vi "XYStage.TestLauncher.vi"() -> ()   [LabVIEW 2017, in "XYStage.lvclass"]
doc: "JKI State Machine Objects (SMO) 1.0.0.5\nJKI - JKI\nCopyright (c) 2016, JKI"
uses:
  XYStage.lvclass
  Typedefs/Coordinates.Units--Cluster.ctl
  Typedefs/Coordinates--Cluster.ctl
  Typedefs/Coordinates.Counts--Cluster.ctl
  XYStage.KIM101/XYStage.KIM101.lvclass
  D:/Program Files (x86)/National Instruments/LabVIEW 2017/vi.lib/JKI/JKI SMO/SMO/SMO.lvclass
  D:/upwork/Laser Measurement Tool/Laser/project/Subsystems/XYStage/XYStage.lvclass
  D:/upwork/Laser Measurement Tool/Laser/project/Subsystems/Device/Device.lvclass
  Typedefs/Configuration--Cluster.ctl
  <vilib>/JKI/JKI SMO/SMO/Typedefs/SMOState --Enum.ctl
  <vilib>/JKI/JKI SMO/SMO/SMO.lvclass
  Device/Device.lvclass
panel:
  out "Move Completed":bool
  out "Current Coordinates":T1
  in  "Wait Timeout, ms":i32=60000
  out "Move Started":bool
  out "Target Coordinates":T1
  in  "Move Absolute":bool
  in  "Units":T2
  out "Init Result":bool
  in  "Y Axis":string="Channel 2"
  in  "X Axis":string="Channel 1"
  in  "Serial Number":string="97000001"
  in  "Home":bool
  out "error out":errorcluster
  in  "Stop":bool
  # "XYStage Test Launcher"
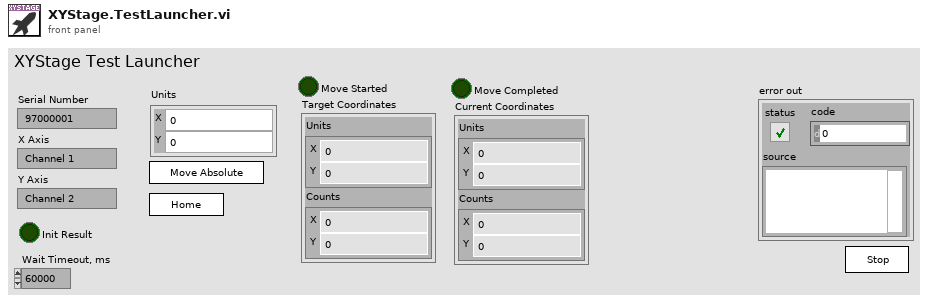
[diagram p1: front panel]
types:
  T1 = typedef "XYStage.lvclass/Coordinates--Cluster.ctl" = cluster{"Units":T2, "Counts":T3}
  T2 = typedef "XYStage.lvclass/Coordinates.Units--Cluster.ctl" = cluster{"X":dbl, "Y":dbl}
  T3 = typedef "XYStage.lvclass/Coordinates.Counts--Cluster.ctl" = cluster{"X":i32, "Y":i32}
  T4 = typedef "XYStage.lvclass/Configuration--Cluster.ctl" = cluster{"Serial Number":string, "X Axis":string, "Y Axis":string, "Real-World Units":string, "Counts per Unit":u32}
  T5 = typedef "XYStage.lvclass/PublicEvents--Cluster.ctl" = cluster{"MoveStarted":refnum<user-event>, "MoveCompleted":refnum<user-event>}
  T6 = typedef "SMO.lvclass/Public Events.ctl" = cluster{"Error":refnum<user-event>, "State":refnum<user-event>, "Reserve State":refnum<user-event>}
  T7 = typedef "SMO.lvclass/SMOState --Enum.ctl" = enum16{"unknown", "Created", "Started", "Stopped"}
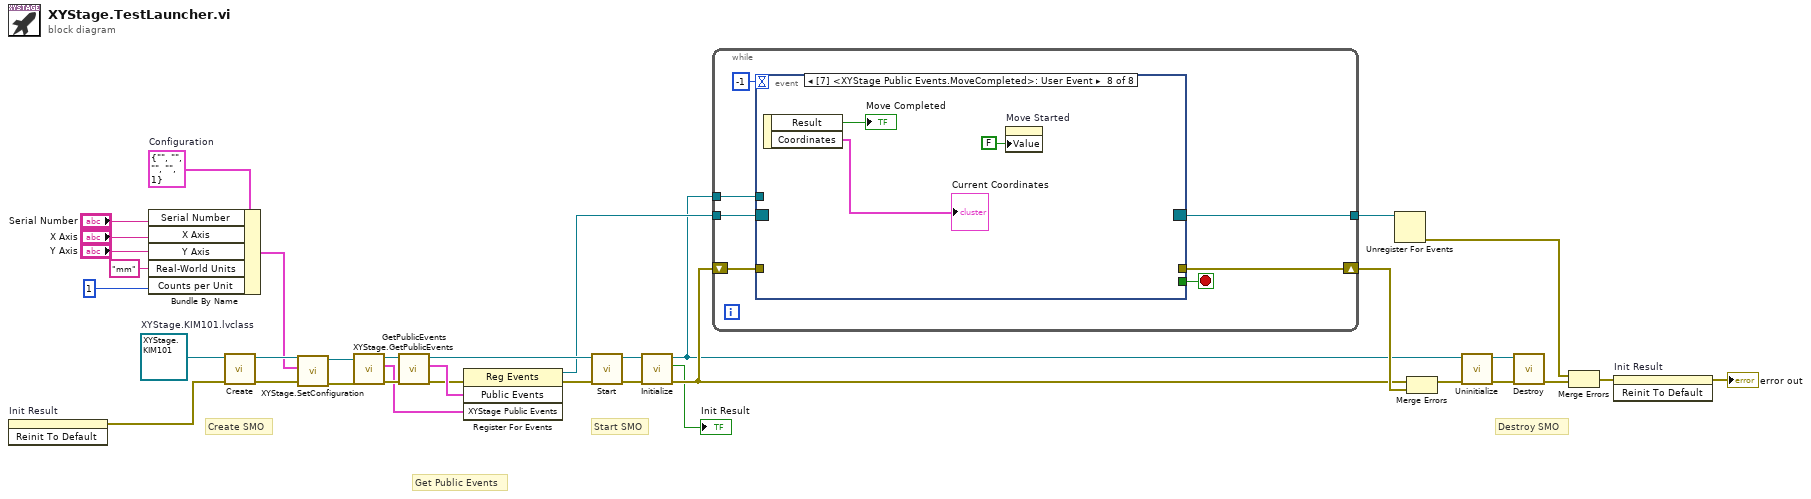
[diagram p0: block diagram]
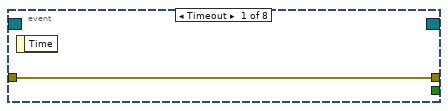
[diagram p2: hidden frame]
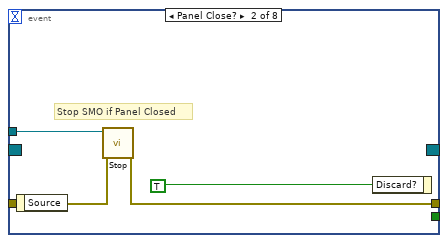
[diagram p3: hidden frame]
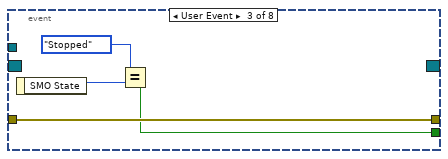
[diagram p4: hidden frame]
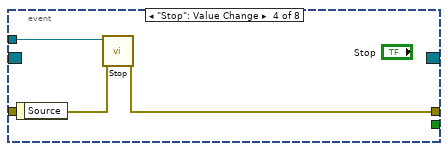
[diagram p5: hidden frame]
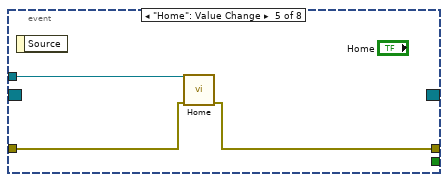
[diagram p6: hidden frame]
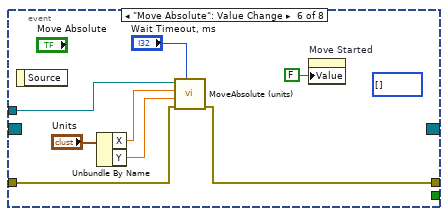
[diagram p7: hidden frame]
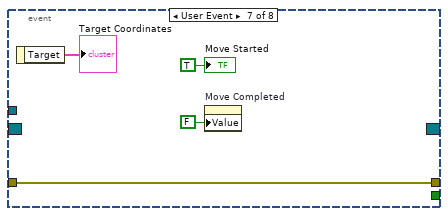
[diagram p8: hidden frame]
diagram:
  w17 = T4 {"Serial Number"="", "X Axis"="", "Y Axis"="", "Real-World Units"="", "Counts per Unit"=1}  # Configuration
  w23 = refnum<class "XYStage.KIM101.lvclass"> refnum  # XYStage.KIM101.lvclass
  # "Get Public Events"
  # "Start SMO"
  # "Destroy SMO"
  # "Create SMO"
  n1 = invoke on="Init Result" class="Bool (strict)" method="Reinit To Default"() -> (error out=w5:errorcluster)  [unwired: 3 in, 2 out]
  n2 = Bundle By Name(cluster=w17, "Serial Number"="Serial Number", "X Axis"="X Axis", "Y Axis"="Y Axis", "Real-World Units"="mm", "Counts per Unit"=u32 1) -> (w18:T4)
  n3 = call <vilib>:"Create.vi"("error in (no error)"=w5, "SMO"=w23) -> ("error out"=w21:errorcluster, "SMO out"=w22:refnum<class "XYStage.KIM101.lvclass">)  [unwired: 7 in, 1 out]
  n4 = call "XYStage.SetConfiguration.vi"("error in (no error)"=w21, "Configuration"=w18, "XYStage"=w22) -> ("error out"=w20:errorcluster, "XYStage out"=w19:refnum<class "XYStage.KIM101.lvclass">)  [unwired: 7 in]
  n5 = call "XYStage.GetPublicEvents.vi"("error in (no error)"=w20, "XYStage"=w19) -> ("error out"=w26:errorcluster, "XYStage Public Events"=w24:T5, "XYStage out"=w25:refnum<class "XYStage.KIM101.lvclass">)  [unwired: 7 in]
  n6 = call <vilib>:"GetPublicEvents.vi"("error in (no error)"=w26, "SMO"=w25) -> ("error out"=w28:errorcluster, "Public Events"=w29:T6, "SMO out"=w31:refnum<class "XYStage.KIM101.lvclass">)  [unwired: 7 in]
  n7 = register-events(error in=w28, w29, w24) -> (reference out=w27:refnum<event-registration>, error out=w30:errorcluster)  [unwired: 1 in]
  n8 = call <vilib>:"Start.vi"("error in (no error)"=w30, "SMO"=w31) -> ("error out"=w12:errorcluster, "SMO out"=w13:refnum<class "XYStage.KIM101.lvclass">)  [unwired: 8 in]
  n9 = call "Initialize.vi"("error in (no error)"=w12, "Device in"=w13) -> ("error out"=w11:errorcluster, "Result"=→"Init Result":bool, "Device out"=w10:refnum<class "XYStage.KIM101.lvclass">)  [unwired: 7 in]
  n10 = while {
    shift-right: [w41] -> w34
    shift-left: w11 -> [w40]
    tunnel: w27 -> [w39]
    tunnel: [w38] -> w35
    tunnel: w10 -> [w37]
    stop <- w42 stop-if-true
    n11 = event shown="[7] <XYStage Public Events.MoveCompleted>: User Event" {
      selector: w39 -> [_ _ _ _ _ _ _ _]
      dyn-events: [_ _ _ _ _ _ _ _] -> w38
      timeout: -1 -> [_ _ _ _ _ _ _ _]
      tunnel: [_ _ w48 _ _ _ _ _] -> w42
      tunnel: w37 -> [_ w47 _ w54 w57 w59 _ _]
      tunnel: [w43 w46 w51 w53 w55 w60 w67 _] -> w41
      tunnel: w40 -> [w43 w45 w51 w52 w56 w61 w67 _]
      event Timeout {
        n12 = event-data() -> ()  [unwired: 1 in, 1 out]
      }
      event Panel Close? {
        # "Stop SMO if Panel Closed"
        n13 = event-data() -> ()  [unwired: 1 in, 1 out]
        n14 = call <vilib>:"Stop.vi"("error in (no error)"=w45, "SMO"=w47) -> ("error out"=w46:errorcluster)  [unwired: 8 in, 1 out]
        n15 = event-data("Discard?"=TRUE ("OK")) -> ()  [unwired: 1 in, 1 out]
      }
      event User Event {
        n16 = event-data() -> ("SMO State"=w50:T7)  [unwired: 1 in]
        n17 = Equal?(x=SMOState_--Enum."Stopped", y=w50) -> (x = y?=w48:bool)
      }
      event "Stop": Value Change {
        n18 = event-data() -> ()  [unwired: 1 in, 1 out]
        n19 = call <vilib>:"Stop.vi"("error in (no error)"=w52, "SMO"=w54) -> ("error out"=w53:errorcluster)  [unwired: 8 in, 1 out]
      }
      event "Home": Value Change {
        n20 = event-data() -> ()  [unwired: 1 in, 1 out]
        n21 = call "Home.vi"("error in (no error)"=w56, "XYStage in"=w57) -> ("error out"=w55:errorcluster)  [unwired: 8 in, 1 out]
      }
      event "Move Absolute": Value Change {
        (unwired) i32[] []
        n22 = event-data() -> ()  [unwired: 1 in, 1 out]
        n23 = Unbundle By Name("Units") -> ("X"=w63:dbl, "Y"=w62:dbl)
        n24 = call "MoveAbsolute (units).vi"("Wait Timeout, ms (60000)"="Wait Timeout, ms", "error in (no error)"=w61, "Y, units"=w62, "X, units"=w63, "XYStage"=w59) -> ("error out"=w60:errorcluster)  [unwired: 5 in, 1 out]
        n25 = property on="Move Started" class="Bool (strict)"("Value"=FALSE ("Move Started")) -> ()  [unwired: 2 in, 2 out]
      }
      event User Event {
        n26 = event-data() -> ("Target"=→"Target Coordinates":T1)  [unwired: 1 in]
        n27 = property on="Move Completed" class="Bool (strict)"("Value"=FALSE ("Move Completed")) -> ()  [unwired: 2 in, 2 out]
        "Move Started" <- TRUE ("Move Started")
      }
      event User Event {
        n28 = event-data() -> ("Result"=→"Move Completed":bool, "Coordinates"=→"Current Coordinates":T1)  [unwired: 1 in]
        n29 = property on="Move Started" class="Bool (strict)"("Value"=FALSE ("Move Started")) -> ()  [unwired: 2 in, 2 out]
      }
    }
  }
  n30 = Unregister For Events(event registration refnum=w35) -> (error out=w33:errorcluster)  [unwired: 1 in]
  n31 = Merge Errors(w11, w34) -> (w8:errorcluster)
  n32 = call "Uninitialize.vi"("error in (no error)"=w8, "Device in"=w10) -> ("error out"=w7:errorcluster, "Device out"=w9:refnum<class "XYStage.KIM101.lvclass">)  [unwired: 8 in]
  n33 = call <vilib>:"Destroy.vi"("error in (no error)"=w7, "SMO"=w9) -> ("error out"=w32:errorcluster)  [unwired: 9 in]
  n34 = Merge Errors(w33, w32) -> (w4:errorcluster)
  n35 = invoke on="Init Result" class="Bool (strict)" method="Reinit To Default"(error in=w4) -> (error out=→"error out":errorcluster)  [unwired: 2 in, 2 out]
